vi "Eagle_FPGA Scanner Control_Micha.vi"() -> ()   [LabVIEW 2015]
uses:
  <vilib>/Platform/TimedLoop/XDataNode/timing_clust.ctl
  <vilib>/Platform/TimedLoop/XDataNode/nitl_modes.ctl
  <vilib>/Platform/TimedLoop/XDataNode/wakeup.ctl
  <vilib>/rvi/Emulation/niFpgaGetClockAttributes.vi
  <vilib>/rvi/Emulation/niFpgaSctlEmulationGetInTimedLoop.vi
  <vilib>/rvi/Emulation/niFpgaEmulationReportErrorSimple.vi
  <vilib>/rvi/eio/common/nirviEmuTemplateMethod_errors.vi
  <vilib>/rvi/Emulation/niFpgaProcessEmulError.vi
  <vilib>/rvi/Emulation/niFpgaCriticalErrorInLSC.vi
  <vilib>/rvi/FXPMathLib/FxpMul/XNode/nifxpmath_Multiplier.xnode
  <vilib>/eio/EIONode/EIONode.xnode
  <vilib>/rvi/FXPMathLib/FxpAdd/XNode/nifxpmath_Add.xnode
  <vilib>/Platform/TimedLoop/XDataNode/XDataNode.xnode
  <vilib>/rvi/FXPMathLib/sim/FxpSim.dll
  <vilib>/Platform/TimedLoop/XDataNode/XDNodeRunTimeDep.lvlib
panel:
  out "Tmp Sens 2":fxp<+,18,3>
  out "Tmp Sens 1":fxp<+,18,3>
  out "X READ 2":fxp<+/-,20,5>
  out "Y READ 2":fxp<+/-,20,5>
  in  "Aim Ctrl":fxp<+,16,3>
  in  "V Range Ctrl":fxp<+,16,3>
  in  "H Range Ctrl":fxp<+,16,3>
  in  "Red Dots Ctrl":fxp<+,16,3>
  in  "LED Ring Ctrl":fxp<+,16,3>
  in  "Y Servo Ena":fxp<+,16,3>
  in  "X Servo Ena":fxp<+,16,3>
  in  "Manual VY":fxp<+/-,20,5>
  in  "Manual VX":fxp<+/-,20,5>
  in  "VX OFFS":fxp<+/-,20,5>
  in  "VY OFFS":fxp<+/-,20,5>
  out "X CMD IND":fxp<+/-,20,5>
  out "Y CMD IND":fxp<+/-,20,5>
  in  "Manual":bool
  in  "NoOfPoints":u16=100
  in  "ScanRate":u32
  in  "NumOfRetries":u16
  out "VX CMD":fxp<+/-,32,17>
  out "VY CMD":fxp<+/-,32,17>
  out "SCAN ENA":bool
  in  "Y Array":fxp<+/-,20,5>[](array[numeric])=[0.0, 0.0, 0.0, 0.0, 0.0, 0.0, 0.0, 0.0, 0.0, 0.0, 0.0, 0.0, 0.0, 0.0, 0.0, 0.0, 0.0, 0.0, 0.0, 0.0, 0.0, 0.0, 0.0, 0.0, 0.0, 0.0, 0.0, 0.0, 0.0, 0.0, 0.0, 0.0, 0.0, 0.0, 0.0, 0.0, 0.0, 0.0, 0.0, 0.0, 0.0, 0.0, 0.0, 0.0, 0.0, 0.0, 0.0, 0.0, 0.0, 0.0, 0.0, 0.0, 0.0, 0.0, 0.0, 0.0, 0.0, 0.0, 0.0, 0.0, 0.0, 0.0, 0.0, 0.0, 0.0, 0.0, 0.0, 0.0, 0.0, 0.0, 0.0, 0.0, 0.0, 0.0, 0.0, 0.0, 0.0, 0.0, 0.0, 0.0, 0.0, 0.0, 0.0, 0.0, 0.0, 0.0, 0.0, 0.0, 0.0, 0.0, 0.0, 0.0, 0.0, 0.0, 0.0, 0.0, 0.0, 0.0, 0.0, 0.0]
  in  "X Array":fxp<+/-,20,5>[](array[numeric])=[0.0, 0.0, 0.0, 0.0, 0.0, 0.0, 0.0, 0.0, 0.0, 0.0, 0.0, 0.0, 0.0, 0.0, 0.0, 0.0, 0.0, 0.0, 0.0, 0.0, 0.0, 0.0, 0.0, 0.0, 0.0, 0.0, 0.0, 0.0, 0.0, 0.0, 0.0, 0.0, 0.0, 0.0, 0.0, 0.0, 0.0, 0.0, 0.0, 0.0, 0.0, 0.0, 0.0, 0.0, 0.0, 0.0, 0.0, 0.0, 0.0, 0.0, 0.0, 0.0, 0.0, 0.0, 0.0, 0.0, 0.0, 0.0, 0.0, 0.0, 0.0, 0.0, 0.0, 0.0, 0.0, 0.0, 0.0, 0.0, 0.0, 0.0, 0.0, 0.0, 0.0, 0.0, 0.0, 0.0, 0.0, 0.0, 0.0, 0.0, 0.0, 0.0, 0.0, 0.0, 0.0, 0.0, 0.0, 0.0, 0.0, 0.0, 0.0, 0.0, 0.0, 0.0, 0.0, 0.0, 0.0, 0.0, 0.0, 0.0]
  in  "Reset":bool
  out "Manual Y IND":fxp<+/-,20,5>
  out "Manual X IND":fxp<+/-,20,5>
  out "Y Servo Rdy":fxp<+,18,3>
  out "X Servo Rdy":fxp<+,18,3>
  out "Y READ":fxp<+/-,20,5>
  out "X READ":fxp<+/-,20,5>
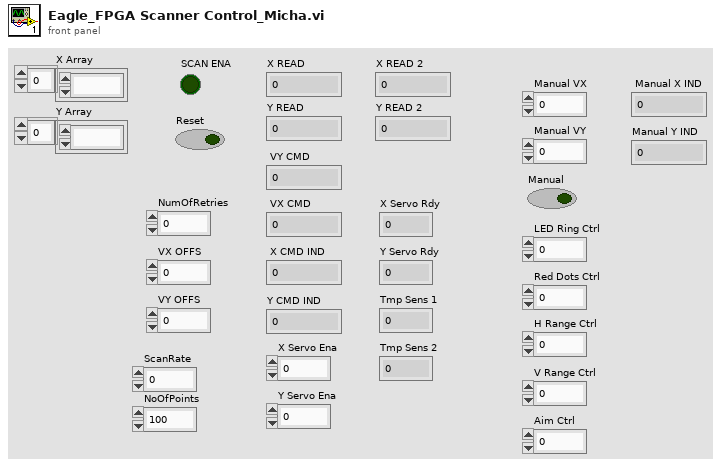
[diagram p1: front panel]
types:
  T1 = typedef "XDNodeRunTimeDep.lvlib/timing_clust.ctl" = cluster{"Expected End [f-1]":u64, "Actual End [f-1]":u64, "Finished Late? [f-1]":bool, "Expected End [i-1]":u64, "Actual End [i-1]":u64, "Finished Late? [i-1]":bool, "Expected Start [i]":u64, "Actual Start [i]":u64, "Expected Start [f]":u64, "Actual Start [f]":u64, "Source Name":string, "Structure Name":string, "Period":i64, "Deadline":i64, "Offset":i64, "Start":i64, "Priority":i32, "Timeout":i32, "Mode":T2, "Wakeup Reason":T3, "Error":errorcluster, "Source Type":string, "Secondary Source Type":string, "Global End Time":u64, "Global Start Time":u64, "Frame Duration":u64, "Iteration Duration":u64, "Assigned CPU":i32, "I/O Scan Engine Mode":u32}
  T2 = typedef "XDNodeRunTimeDep.lvlib/nitl_modes.ctl" = enum32{"No Change", "Process missed periods, maintain original phase", "Discard missed periods, maintain original phase", "Process missed periods, ignore original phase", "Discard missed periods, ignore original phase"}
  T3 = typedef "XDNodeRunTimeDep.lvlib/wakeup.ctl" = enum32{"Normal", "Aborted", "Asynchronous wakeup", "Timing source error", "Timed loop error", "Timeout"}
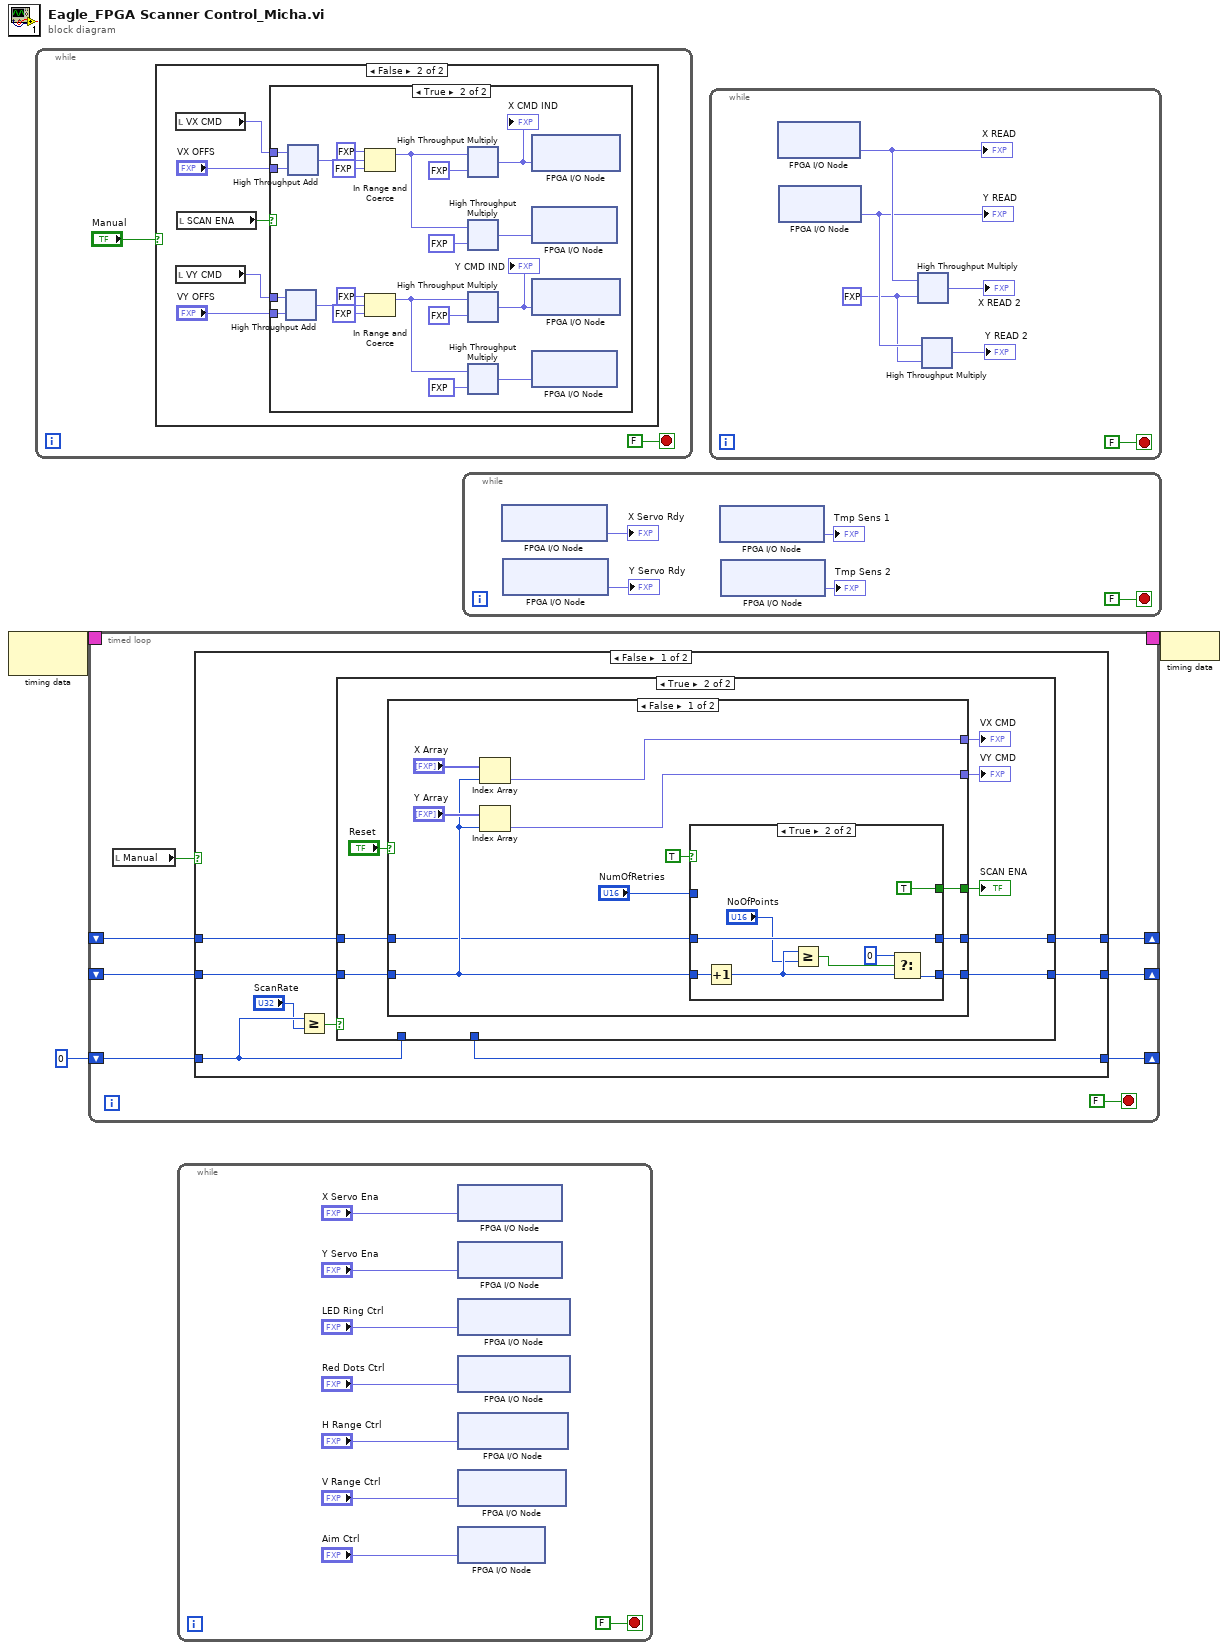
[diagram p0: block diagram]
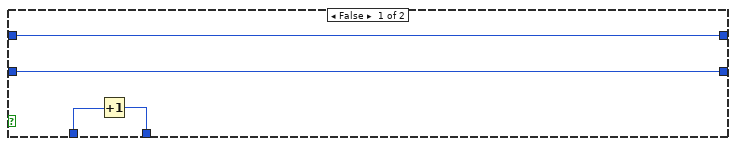
[diagram p2: hidden frame]
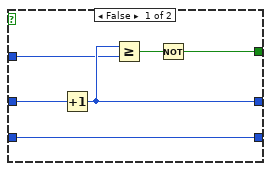
[diagram p3: hidden frame]
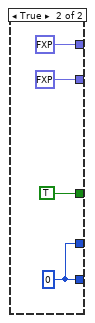
[diagram p4: hidden frame]
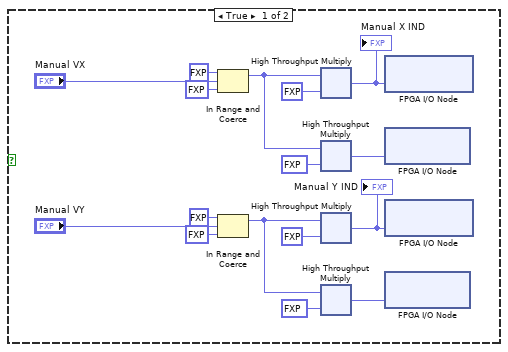
[diagram p6: hidden frame]
diagram:
  n1 = node-c288() -> (w3:T1)  [unwired: 1 in]
  n2 = while {
    stop <- FALSE stop-if-true
    n3 = case shown="False" "Manual" {
      frame True {
        n4 = In Range and Coerce(upper limit=fxp<+/-,20,5> 10.0, x="Manual VX", lower limit=fxp<+/-,20,5> -10.0 ("upper limit")) -> (coerced(x)=w13:fxp<+/-,20,5>)  [unwired: 1 out]
        n5 = In Range and Coerce(upper limit=fxp<+/-,20,5> 10.0, x="Manual VY", lower limit=fxp<+/-,20,5> -10.0 ("upper limit")) -> (coerced(x)=w8:fxp<+/-,20,5>)  [unwired: 1 out]
        n6 = xnode ("High Throughput Multiply")("x"=w13, "y"=fxp<+/-,20,5> 0.5) -> ("x*y"=w19:fxp<+/-,20,5>)
        "Manual X IND" <- w19
        n7 = xnode ("High Throughput Multiply")("x"=w13, "y"=fxp<+/-,20,5> -0.5) -> ("x*y"=w17:fxp<+/-,20,5>)
        n8 = xnode ("High Throughput Multiply")("x"=w8, "y"=fxp<+/-,20,5> 0.5) -> ("x*y"=w15:fxp<+/-,20,5>)
        "Manual Y IND" <- w15
        n9 = xnode ("High Throughput Multiply")("x"=w8, "y"=fxp<+/-,20,5> -0.5) -> ("x*y"=w14:fxp<+/-,20,5>)
        n10 = xnode "FPGA I/O Node"("X CMD+"=w19) -> ()  [unwired: 1 in, 1 out]
        n11 = xnode "FPGA I/O Node"("X CMD-"=w17) -> ()  [unwired: 1 in, 1 out]
        n12 = xnode "FPGA I/O Node"("Y CMD+"=w15) -> ()  [unwired: 1 in, 1 out]
        n13 = xnode "FPGA I/O Node"("Y CMD-"=w14) -> ()  [unwired: 1 in, 1 out]
      }
      frame False {
        n14 = local read "VX CMD"() -> (w23:fxp<+/-,32,17>)
        n15 = local read "VY CMD"() -> (w22:fxp<+/-,32,17>)
        n16 = local read "SCAN ENA"() -> (w24:bool)
        n17 = case shown="True" w24 {
          tunnel: "VX OFFS" -> [_ w38]
          tunnel: "VY OFFS" -> [_ w37]
          tunnel: w23 -> [_ w28]
          tunnel: w22 -> [_ w27]
          frame False {
          }
          frame True {
            n18 = xnode ("High Throughput Add")("x"=w27, "y"=w37) -> ("x+y"=w30:fxp<+/-,33,18>)
            n19 = xnode ("High Throughput Add")("x"=w28, "y"=w38) -> ("x+y"=w36:fxp<+/-,33,18>)
            n20 = In Range and Coerce(upper limit=fxp<+/-,20,5> 10.0, x=w36, lower limit=fxp<+/-,20,5> -10.0 ("upper limit")) -> (coerced(x)=w35:fxp<+/-,33,18>)  [unwired: 1 out]
            n21 = In Range and Coerce(upper limit=fxp<+/-,20,5> 10.0, x=w30, lower limit=fxp<+/-,20,5> -10.0 ("upper limit")) -> (coerced(x)=w29:fxp<+/-,33,18>)  [unwired: 1 out]
            n22 = xnode ("High Throughput Multiply")("x"=w35, "y"=fxp<+/-,20,5> 0.5) -> ("x*y"=w44:fxp<+/-,20,5>)
            "X CMD IND" <- w44
            n23 = xnode ("High Throughput Multiply")("x"=w35, "y"=fxp<+/-,20,5> -0.5) -> ("x*y"=w42:fxp<+/-,20,5>)
            n24 = xnode ("High Throughput Multiply")("x"=w29, "y"=fxp<+/-,20,5> 0.5) -> ("x*y"=w40:fxp<+/-,20,5>)
            "Y CMD IND" <- w40
            n25 = xnode ("High Throughput Multiply")("x"=w29, "y"=fxp<+/-,20,5> -0.5) -> ("x*y"=w39:fxp<+/-,20,5>)
            n26 = xnode "FPGA I/O Node"("X CMD+"=w44) -> ()  [unwired: 1 in, 1 out]
            n27 = xnode "FPGA I/O Node"("X CMD-"=w42) -> ()  [unwired: 1 in, 1 out]
            n28 = xnode "FPGA I/O Node"("Y CMD+"=w40) -> ()  [unwired: 1 in, 1 out]
            n29 = xnode "FPGA I/O Node"("Y CMD-"=w39) -> ()  [unwired: 1 in, 1 out]
          }
        }
      }
    }
  }
  n30 = timed-loop {
    timing: w3 -> [_]
    timing-out: [_] -> w2
    shift-right: [w50] -> _
    shift-left: _ -> [w53]
    shift-right: [w52] -> _
    shift-left: _ -> [w51]
    shift-right: [w49] -> _
    shift-left: u32 0 -> [w48]
    stop <- FALSE stop-if-true
    n31 = local read "Manual"() -> (w47:bool)
    n32 = case shown="False" w47 {
      tunnel: w53 -> [w62 w105]
      tunnel: [w61 w106] -> w52
      tunnel: w51 -> [w60 w106]
      tunnel: [w59 w105] -> w50
      tunnel: [w57 w104] -> w49
      tunnel: w48 -> [w56 w104]
      frame False {
        n33 = Greater Or Equal?(x=w56, y="ScanRate") -> (x >= y?=w58:bool)
        n34 = case shown="True" w58 {
          tunnel: w62 -> [w65 w73]
          tunnel: [w66 w69] -> w61
          tunnel: w60 -> [w66 w68]
          tunnel: [w65 w67] -> w59
          tunnel: w56 -> [w64 _]
          tunnel: [w63 _] -> w57
          frame False {
            n35 = Increment(x=w64) -> (x+1=w63:u32)
          }
          frame True {
            n36 = case shown="False" "Reset" {
              tunnel: w73 -> [w83 _]
              tunnel: [w76 fxp<+/-,20,5> 10.0 ("VX CMD")] -> w72
              tunnel: [w75 fxp<+/-,20,5> 10.0 ("VY CMD")] -> w71
              tunnel: [w78 TRUE ("SCAN ENA")] -> w70
              tunnel: [w80 w100] -> w69
              tunnel: w68 -> [w81 _]
              tunnel: [w82 w100] -> w67
              frame False {
                n37 = Index Array(array="X Array", index=w83) -> (element=w76:fxp<+/-,20,5>)
                n38 = Index Array(array="Y Array", index=w83) -> (element=w75:fxp<+/-,20,5>)
                n39 = case shown="True" TRUE {
                  tunnel: w83 -> [w91 w99]
                  tunnel: [w91 w96] -> w82
                  tunnel: w81 -> [w90 w97]
                  tunnel: [w89 w97] -> w80
                  tunnel: "NumOfRetries" -> [w88 _]
                  tunnel: [w86 TRUE] -> w78
                  frame False {
                    n40 = Increment(x=w90) -> (x+1=w89:u16)
                    n41 = Greater Or Equal?(x=w89, y=w88) -> (x >= y?=w87:bool)
                    n42 = Not(x=w87) -> (.not. x?=w86:bool)
                  }
                  frame True {
                    n43 = Increment(x=w99) -> (x+1=w94:u16)
                    n44 = Greater Or Equal?(x=w94, y="NoOfPoints") -> (x >= y?=w92:bool)
                    n45 = Select(t=u16 0, s=w92, f=w94) -> (s? t:f=w96:u16)
                  }
                }
              }
              frame True {
                w100 = u16 0
              }
            }
            "SCAN ENA" <- w70
            "VY CMD" <- w71
            "VX CMD" <- w72
          }
        }
      }
      frame True {
      }
    }
  }
  n46 = while {
    stop <- FALSE stop-if-true
    n47 = xnode "FPGA I/O Node"("X Servo Ena"="X Servo Ena") -> ()  [unwired: 1 in, 1 out]
    n48 = xnode "FPGA I/O Node"("Y Servo Ena"="Y Servo Ena") -> ()  [unwired: 1 in, 1 out]
    n49 = xnode "FPGA I/O Node"("LED Ring Ctrl"="LED Ring Ctrl") -> ()  [unwired: 1 in, 1 out]
    n50 = xnode "FPGA I/O Node"("Red Dots Ctrl"="Red Dots Ctrl") -> ()  [unwired: 1 in, 1 out]
    n51 = xnode "FPGA I/O Node"("H Range Ctrl"="H Range Ctrl") -> ()  [unwired: 1 in, 1 out]
    n52 = xnode "FPGA I/O Node"("V Range Ctrl"="V Range Ctrl") -> ()  [unwired: 1 in, 1 out]
    n53 = xnode "FPGA I/O Node"("Aim Ctrl"="Aim Ctrl") -> ()  [unwired: 1 in, 1 out]
  }
  n54 = while {
    stop <- FALSE stop-if-true
    n55 = xnode "FPGA I/O Node"() -> ("X Servo Rdy"=→"X Servo Rdy":fxp<+,18,3>)  [unwired: 1 in, 1 out]
    n56 = xnode "FPGA I/O Node"() -> ("Y Servo Rdy"=→"Y Servo Rdy":fxp<+,18,3>)  [unwired: 1 in, 1 out]
    n57 = xnode "FPGA I/O Node"() -> ("Tmp Sens 1"=→"Tmp Sens 1":fxp<+,18,3>)  [unwired: 1 in, 1 out]
    n58 = xnode "FPGA I/O Node"() -> ("Tmp Sens 2"=→"Tmp Sens 2":fxp<+,18,3>)  [unwired: 1 in, 1 out]
  }
  n59 = while {
    stop <- FALSE stop-if-true
    w122 = fxp<+/-,20,5> 2.0 ("Y READ")
    n60 = xnode "FPGA I/O Node"() -> ("X READ"=w124:fxp<+/-,20,5>)  [unwired: 1 in, 1 out]
    "X READ" <- w124
    n61 = xnode "FPGA I/O Node"() -> ("Y READ"=w123:fxp<+/-,20,5>)  [unwired: 1 in, 1 out]
    "Y READ" <- w123
    n62 = xnode ("High Throughput Multiply")("x"=w124, "y"=w122) -> ("x*y"=→"X READ 2":fxp<+/-,20,5>)
    n63 = xnode ("High Throughput Multiply")("x"=w123, "y"=w122) -> ("x*y"=→"Y READ 2":fxp<+/-,20,5>)
  }
  n64 = node-c288(w2) -> ()
